vi "Drivetrain Control.vi"(0 "Back Left DevRef In":T1={"DeviceStatus"={"status"=FALSE, "code"=0, "source"=""}, "Type"=enum."PWM", "PWM"={"Digital Module"=enum."Digital Module 1", "PWM Channel"=enum."Invalid", "DeadBand"={"Name"="", "maxPositivePwm"=0, "minPositivePwm"=0, "centerPwm"=0, "maxNegativePwm"=0, "minNegativePwm"=0, "angularRange"=0}}, "CAN"={"Device Number"=0, "Control Mode"=enum."Percent VBus", "Semaphore"=refnum, "Max Vout"=12.0}, "Invert"=FALSE, "TransformRef"=refnum, "InvTransformRef"=refnum}, 1 "X Axis":dbl, 2 "Y Axis":dbl, 5 "Back Right DevRef In":T1={"DeviceStatus"={"status"=FALSE, "code"=0, "source"=""}, "Type"=enum."PWM", "PWM"={"Digital Module"=enum."Digital Module 1", "PWM Channel"=enum."Invalid", "DeadBand"={"Name"="", "maxPositivePwm"=0, "minPositivePwm"=0, "centerPwm"=0, "maxNegativePwm"=0, "minNegativePwm"=0, "angularRange"=0}}, "CAN"={"Device Number"=0, "Control Mode"=enum."Percent VBus", "Semaphore"=refnum, "Max Vout"=12.0}, "Invert"=FALSE, "TransformRef"=refnum, "InvTransformRef"=refnum}, 7 "Front Left DevRef In":T1={"DeviceStatus"={"status"=FALSE, "code"=0, "source"=""}, "Type"=enum."PWM", "PWM"={"Digital Module"=enum."Digital Module 1", "PWM Channel"=enum."Invalid", "DeadBand"={"Name"="", "maxPositivePwm"=0, "minPositivePwm"=0, "centerPwm"=0, "maxNegativePwm"=0, "minNegativePwm"=0, "angularRange"=0}}, "CAN"={"Device Number"=0, "Control Mode"=enum."Percent VBus", "Semaphore"=refnum, "Max Vout"=12.0}, "Invert"=FALSE, "TransformRef"=refnum, "InvTransformRef"=refnum}, 9 "Front Right DevRef In":T1={"DeviceStatus"={"status"=FALSE, "code"=0, "source"=""}, "Type"=enum."PWM", "PWM"={"Digital Module"=enum."Digital Module 1", "PWM Channel"=enum."Invalid", "DeadBand"={"Name"="", "maxPositivePwm"=0, "minPositivePwm"=0, "centerPwm"=0, "maxNegativePwm"=0, "minNegativePwm"=0, "angularRange"=0}}, "CAN"={"Device Number"=0, "Control Mode"=enum."Percent VBus", "Semaphore"=refnum, "Max Vout"=12.0}, "Invert"=FALSE, "TransformRef"=refnum, "InvTransformRef"=refnum}, 11 "Closed Loop On/Off":bool, 12 "Drivetrain Reverse Button":bool, 13 "Trigger":bool) -> (3 "Left Motor Value":dbl, 4 "Back Left DevRef Out":T1={"DeviceStatus"={"status"=FALSE, "code"=0, "source"=""}, "Type"=enum."PWM", "PWM"={"Digital Module"=enum."Digital Module 1", "PWM Channel"=enum."Invalid", "DeadBand"={"Name"="", "maxPositivePwm"=0, "minPositivePwm"=0, "centerPwm"=0, "maxNegativePwm"=0, "minNegativePwm"=0, "angularRange"=0}}, "CAN"={"Device Number"=0, "Control Mode"=enum."Percent VBus", "Semaphore"=refnum, "Max Vout"=12.0}, "Invert"=FALSE, "TransformRef"=refnum, "InvTransformRef"=refnum}, 6 "Back Right DevRef Out":T1={"DeviceStatus"={"status"=FALSE, "code"=0, "source"=""}, "Type"=enum."PWM", "PWM"={"Digital Module"=enum."Digital Module 1", "PWM Channel"=enum."Invalid", "DeadBand"={"Name"="", "maxPositivePwm"=0, "minPositivePwm"=0, "centerPwm"=0, "maxNegativePwm"=0, "minNegativePwm"=0, "angularRange"=0}}, "CAN"={"Device Number"=0, "Control Mode"=enum."Percent VBus", "Semaphore"=refnum, "Max Vout"=12.0}, "Invert"=FALSE, "TransformRef"=refnum, "InvTransformRef"=refnum}, 8 "Front Left DevRef Out":T1={"DeviceStatus"={"status"=FALSE, "code"=0, "source"=""}, "Type"=enum."PWM", "PWM"={"Digital Module"=enum."Digital Module 1", "PWM Channel"=enum."Invalid", "DeadBand"={"Name"="", "maxPositivePwm"=0, "minPositivePwm"=0, "centerPwm"=0, "maxNegativePwm"=0, "minNegativePwm"=0, "angularRange"=0}}, "CAN"={"Device Number"=0, "Control Mode"=enum."Percent VBus", "Semaphore"=refnum, "Max Vout"=12.0}, "Invert"=FALSE, "TransformRef"=refnum, "InvTransformRef"=refnum}, 10 "Front Right DevRef Out":T1={"DeviceStatus"={"status"=FALSE, "code"=0, "source"=""}, "Type"=enum."PWM", "PWM"={"Digital Module"=enum."Digital Module 1", "PWM Channel"=enum."Invalid", "DeadBand"={"Name"="", "maxPositivePwm"=0, "minPositivePwm"=0, "centerPwm"=0, "maxNegativePwm"=0, "minNegativePwm"=0, "angularRange"=0}}, "CAN"={"Device Number"=0, "Control Mode"=enum."Percent VBus", "Semaphore"=refnum, "Max Vout"=12.0}, "Invert"=FALSE, "TransformRef"=refnum, "InvTransformRef"=refnum}, 14 "Right Motor Value":dbl)   [LabVIEW 2012]
uses:
  <vilib>/Rock Robotics/WPI/MotorControl/WPI_MotorControlDeviceRef.ctl
  <vilib>/Rock Robotics/SystemInterfaces/Typedef/FPGA_TypedefDigitalModule.ctl
  <vilib>/Rock Robotics/SystemInterfaces/DIO/FPGA_DIOPWMChannel.ctl
  <vilib>/Rock Robotics/WPI/PWM/WPI_PWMDeadband.ctl
  <vilib>/Rock Robotics/WPI/CAN/Jaguar/SubVIs/WPI_CANJaguar_ControlMode.ctl
  <vilib>/Rock Robotics/WPI/PWM/WPI_PWMTransform_ConPane.ctl
  <vilib>/Rock Robotics/WPI/CAN/Jaguar/SubVIs/WPI_CANJaguar_SpeedReference.ctl
  Robot Global Data.vi
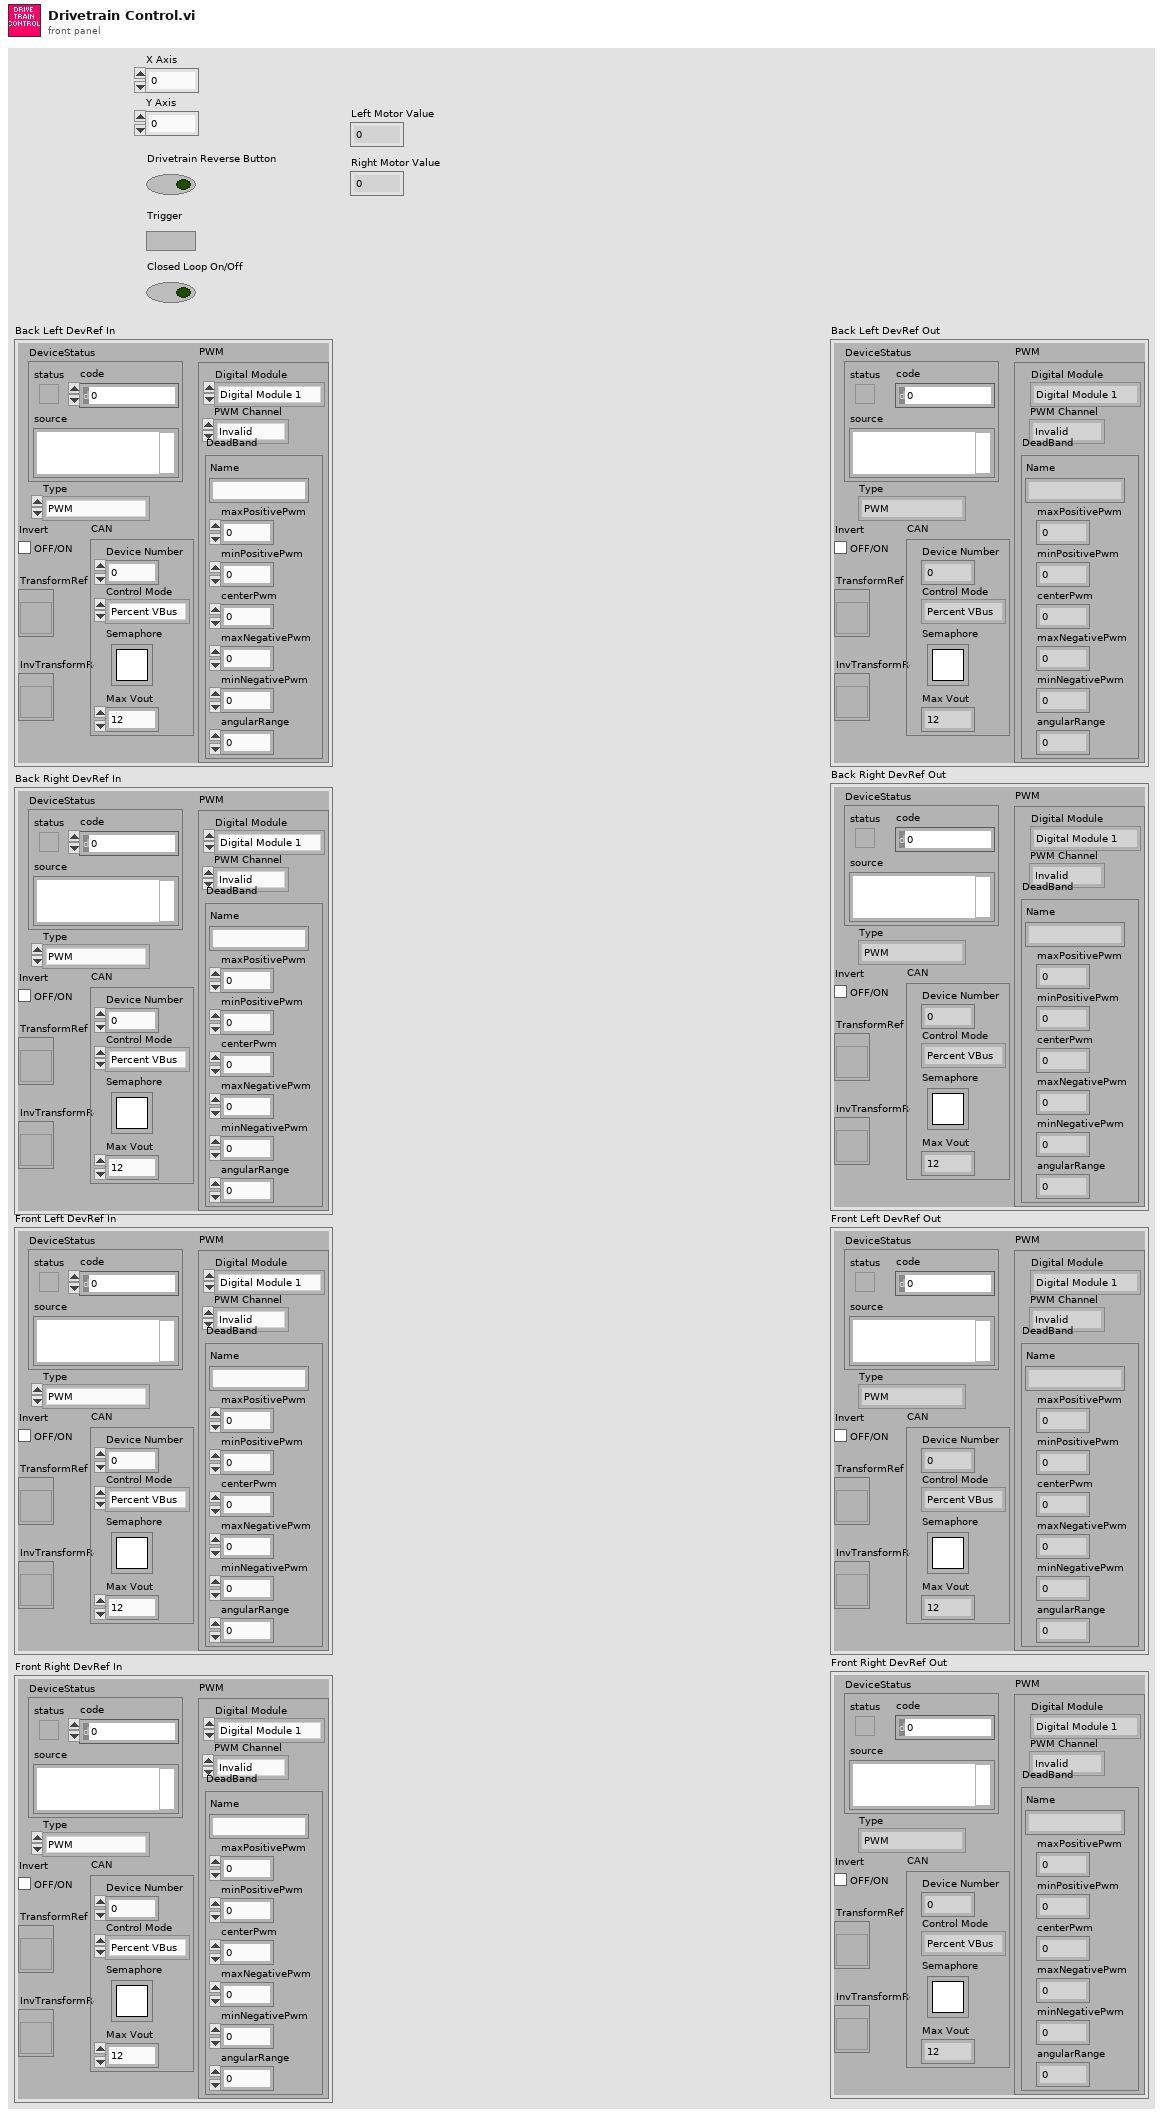
[diagram p1: front panel]
types:
  T1 = typedef "WPI_MotorControlDeviceRef.ctl" = cluster{"DeviceStatus":errorcluster, "Type":enum16{"PWM", "CAN"}, "PWM":cluster{"Digital Module":T2, "PWM Channel":T3, "DeadBand":T4}, "CAN":cluster{"Device Number":u8, "Control Mode":T5, "Semaphore":T6, "Max Vout":dbl}, "Invert":bool, "TransformRef":T7, "InvTransformRef":T7}
  T2 = typedef "FPGA_TypedefDigitalModule.ctl" = enum16{"Digital Module 1", "Digital Module 2"}
  T3 = typedef "FPGA_DIOPWMChannel.ctl" = enum8{"PWM 1", "PWM 2", "PWM 3", "PWM 4", "PWM 5", "PWM 6", "PWM 7", "PWM 8", "PWM 9", "PWM 10", "Invalid"}
  T4 = typedef "WPI_PWMDeadband.ctl" = cluster{"Name":string, "maxPositivePwm":i32, "minPositivePwm":i32, "centerPwm":i32, "maxNegativePwm":i32, "minNegativePwm":i32, "angularRange":u16}
  T5 = typedef "WPI_CANJaguar_ControlMode.ctl" = enum8{"Percent VBus", "Current", "Speed", "Position", "Voltage"}
  T6 = typedef "Semaphore RefNum" = refnum<k1>
  T7 = typedef "WPI_PWMTransform_ConPane.ctl" = refnum<vi>
  T8 = typedef "WPI_CANJaguar_SpeedReference.ctl" = u8
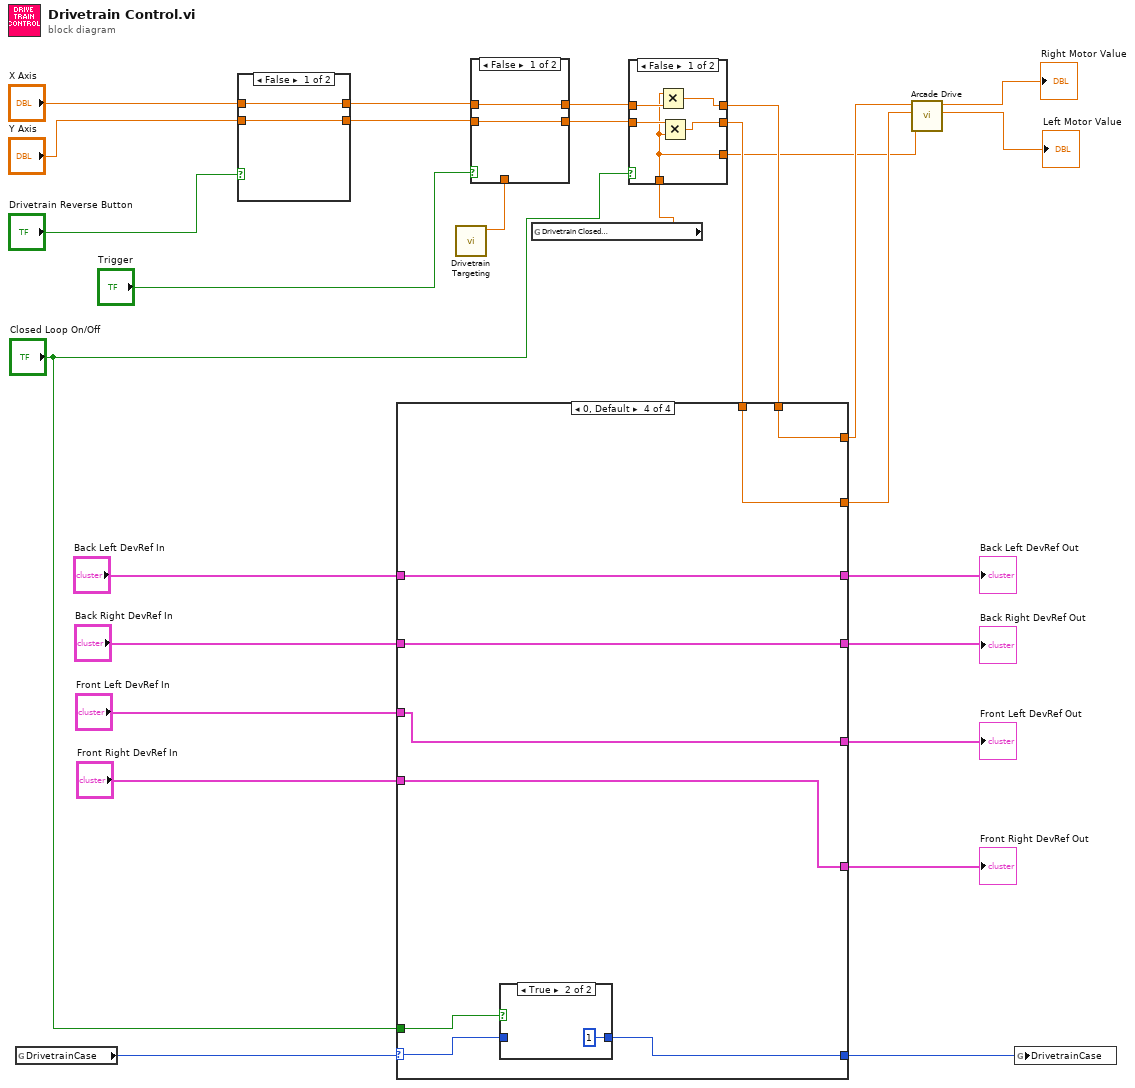
[diagram p0: block diagram]
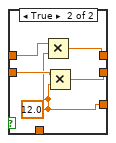
[diagram p2: hidden frame]
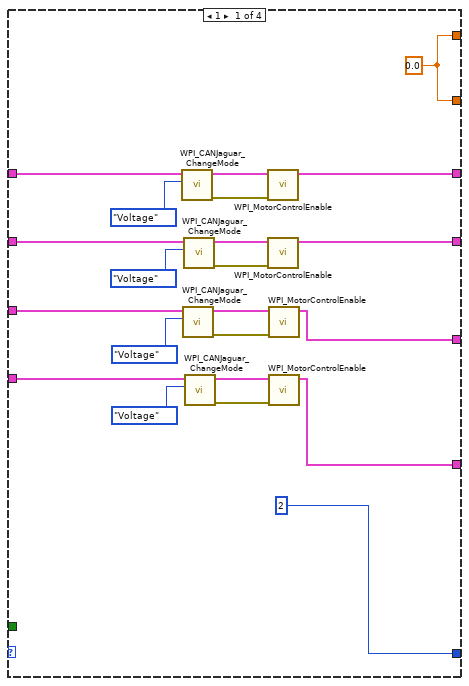
[diagram p3: hidden frame]
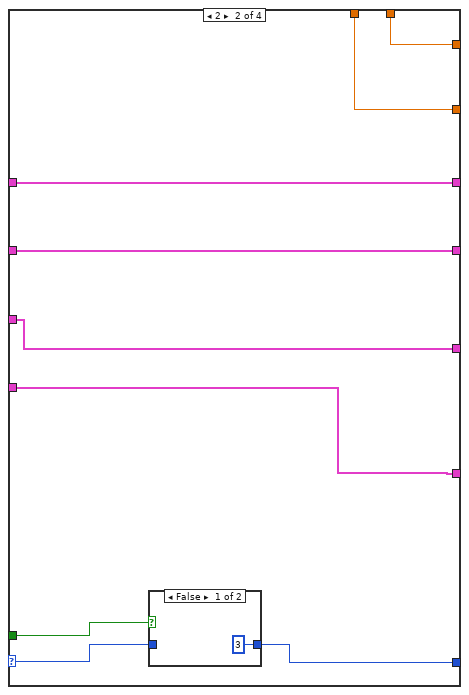
[diagram p4: hidden frame]
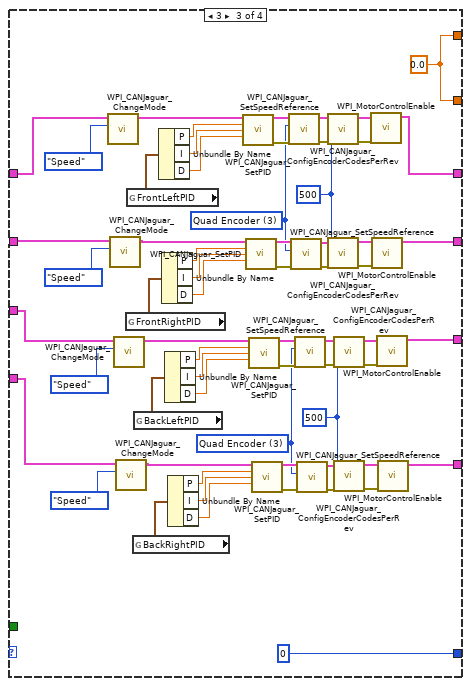
[diagram p6: hidden frame]
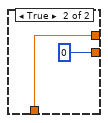
[diagram p8: hidden frame]
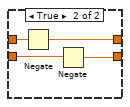
[diagram p9: hidden frame]
diagram:
  n1 = global read "Robot Global Data.vi" "DrivetrainCase"() -> (w20:i8)
  n2 = case shown="False" "Drivetrain Reverse Button" {
    tunnel: [w30 w31] -> w28
    tunnel: "X Axis" -> [w30 w34]
    tunnel: [w29 w32] -> w27
    tunnel: "Y Axis" -> [w29 w33]
    frame False {
    }
    frame True {
      n3 = Negate(x=w34) -> (-x=w31:dbl)
      n4 = Negate(x=w33) -> (-x=w32:dbl)
    }
  }
  n5 = call "Drivetrain Targeting.vi"() -> ("Drivetrain Center"=w23:dbl)  [unwired: 11 in]
  n6 = case shown="False" "Trigger" {
    tunnel: [w36 w37] -> w18
    tunnel: w28 -> [w36 _]
    tunnel: [w35 0] -> w17
    tunnel: w27 -> [w35 _]
    tunnel: w23 -> [_ w37]
    frame False {
    }
    frame True {
    }
  }
  n7 = global read "Robot Global Data.vi" "Drivetrain Closed\nLoop Max"() -> (w16:dbl)
  n8 = case shown="False" "Closed Loop On/Off" {
    tunnel: [w41 w46] -> w14
    tunnel: w18 -> [w43 w48]
    tunnel: [w40 w45] -> w15
    tunnel: w17 -> [w42 w47]
    tunnel: w16 -> [w39 _]
    tunnel: [w39 w44] -> w2
    frame False {
      n9 = Multiply(x=w39, y=w43) -> (x*y=w41:dbl)
      n10 = Multiply(x=w42, y=w39) -> (x*y=w40:dbl)
    }
    frame True {
      w44 = 12.0
      n11 = Multiply(x=w48, y=w44) -> (x*y=w46:dbl)
      n12 = Multiply(x=w47, y=w44) -> (x*y=w45:dbl)
    }
  }
  n13 = case shown="0, Default" w20 {
    selector: w20 -> [_ w76 _ w148]
    tunnel: [i8 2 ("ShooterCase") w75 i8 0 ("ShooterCase") w149] -> w19
    tunnel: "Back Left DevRef In" -> [w69 w79 w141 w152]
    tunnel: "Back Right DevRef In" -> [w68 w78 w140 w151]
    tunnel: [w61 w79 w113 w152] -> w6
    tunnel: [w60 w78 w114 w151] -> w5
    tunnel: "Closed Loop On/Off" -> [_ w77 _ w150]
    tunnel: w14 -> [_ w73 _ w147]
    tunnel: w15 -> [_ w74 _ w146]
    tunnel: [w59 w73 w112 w147] -> w13
    tunnel: [w59 w74 w112 w146] -> w12
    tunnel: "Front Left DevRef In" -> [w52 w72 w85 w145]
    tunnel: "Front Right DevRef In" -> [w51 w71 w84 w144]
    tunnel: [w50 w72 w83 w145] -> w4
    tunnel: [w49 w71 w82 w144] -> w3
    frame 1 {
      w59 = 0.0 ("FSpeed")
      n14 = call <vilib>:"WPI_CANJaguar_ChangeMode.vi"("Control Mode"=WPI_CANJaguar_ControlMode."Voltage", "CAN Jaguar Ref"=w69) -> ("error out"=w62:errorcluster, "CAN Jaguar Ref Out"=w63:T1)  [unwired: 8 in]
      n15 = call <vilib>:"WPI_CANJaguar_ChangeMode.vi"("Control Mode"=WPI_CANJaguar_ControlMode."Voltage", "CAN Jaguar Ref"=w52) -> ("error out"=w53:errorcluster, "CAN Jaguar Ref Out"=w54:T1)  [unwired: 8 in]
      n16 = call <vilib>:"WPI_CANJaguar_ChangeMode.vi"("Control Mode"=WPI_CANJaguar_ControlMode."Voltage", "CAN Jaguar Ref"=w68) -> ("error out"=w64:errorcluster, "CAN Jaguar Ref Out"=w65:T1)  [unwired: 8 in]
      n17 = call <vilib>:"WPI_CANJaguar_ChangeMode.vi"("Control Mode"=WPI_CANJaguar_ControlMode."Voltage", "CAN Jaguar Ref"=w51) -> ("error out"=w55:errorcluster, "CAN Jaguar Ref Out"=w56:T1)  [unwired: 8 in]
      n18 = call <vilib>:"WPI_MotorControlEnable.vi"("error in (no error)"=w62, "CAN Jaguar Ref"=w63) -> ("CAN Jaguar Ref Out"=w61:T1)  [unwired: 8 in, 1 out]
      n19 = call <vilib>:"WPI_MotorControlEnable.vi"("error in (no error)"=w64, "CAN Jaguar Ref"=w65) -> ("CAN Jaguar Ref Out"=w60:T1)  [unwired: 8 in, 1 out]
      n20 = call <vilib>:"WPI_MotorControlEnable.vi"("error in (no error)"=w53, "CAN Jaguar Ref"=w54) -> ("CAN Jaguar Ref Out"=w50:T1)  [unwired: 8 in, 1 out]
      n21 = call <vilib>:"WPI_MotorControlEnable.vi"("error in (no error)"=w55, "CAN Jaguar Ref"=w56) -> ("CAN Jaguar Ref Out"=w49:T1)  [unwired: 8 in, 1 out]
    }
    frame 2 {
      n22 = case shown="False" w77 {
        tunnel: [i8 3 ("ShooterCase") w81] -> w75
        tunnel: w76 -> [_ w81]
        frame False {
        }
        frame True {
        }
      }
    }
    frame 3 {
      w90 = u16 500 ("Encoder Codes Per Rev")
      w95 = T8 3 items=["Encoder"=0, "Inv Encoder"=2, "Quad Encoder"=3, "None"=255] ("Speed Reference")
      w112 = 0.0 ("FSpeed")
      w119 = u16 500 ("Encoder Codes Per Rev")
      w124 = T8 3 items=["Encoder"=0, "Inv Encoder"=2, "Quad Encoder"=3, "None"=255] ("Speed Reference")
      n23 = call <vilib>:"WPI_CANJaguar_ChangeMode.vi"("Control Mode"=WPI_CANJaguar_ControlMode."Speed", "CAN Jaguar Ref"=w141) -> ("CAN Jaguar Ref Out"=w139:T1)  [unwired: 8 in, 1 out]
      n24 = call <vilib>:"WPI_CANJaguar_ChangeMode.vi"("Control Mode"=WPI_CANJaguar_ControlMode."Speed", "CAN Jaguar Ref"=w140) -> ("CAN Jaguar Ref Out"=w130:T1)  [unwired: 8 in, 1 out]
      n25 = call <vilib>:"WPI_CANJaguar_ChangeMode.vi"("Control Mode"=WPI_CANJaguar_ControlMode."Speed", "CAN Jaguar Ref"=w85) -> ("CAN Jaguar Ref Out"=w109:T1)  [unwired: 8 in, 1 out]
      n26 = call <vilib>:"WPI_CANJaguar_ChangeMode.vi"("Control Mode"=WPI_CANJaguar_ControlMode."Speed", "CAN Jaguar Ref"=w84) -> ("CAN Jaguar Ref Out"=w100:T1)  [unwired: 8 in, 1 out]
      n27 = global read "Robot Global Data.vi" "FrontRightPID"() -> (w134:cluster{"P":dbl, "I":dbl, "D":dbl})
      n28 = global read "Robot Global Data.vi" "FrontLeftPID"() -> (w138:cluster{"P":dbl, "I":dbl, "D":dbl})
      n29 = global read "Robot Global Data.vi" "BackRightPID"() -> (w104:cluster{"P":dbl, "I":dbl, "D":dbl})
      n30 = global read "Robot Global Data.vi" "BackLeftPID"() -> (w108:cluster{"P":dbl, "I":dbl, "D":dbl})
      n31 = Unbundle By Name(w138) -> ("P"=w137:dbl, "I"=w136:dbl, "D"=w135:dbl)
      n32 = Unbundle By Name(w134) -> ("P"=w133:dbl, "I"=w132:dbl, "D"=w131:dbl)
      n33 = Unbundle By Name(w108) -> ("P"=w107:dbl, "I"=w106:dbl, "D"=w105:dbl)
      n34 = Unbundle By Name(w104) -> ("P"=w103:dbl, "I"=w102:dbl, "D"=w101:dbl)
      n35 = call <vilib>:"WPI_CANJaguar_SetPID.vi"("CAN Jaguar Ref"=w139, "P"=w137, "I"=w136, "D"=w135) -> ("CAN Jaguar Ref Out"=w127:T1, "error out"=w128:errorcluster)  [unwired: 10 in]
      n36 = call <vilib>:"WPI_CANJaguar_SetPID.vi"("CAN Jaguar Ref"=w130, "P"=w133, "I"=w132, "D"=w131) -> ("CAN Jaguar Ref Out"=w126:T1, "error out"=w125:errorcluster)  [unwired: 10 in]
      n37 = call <vilib>:"WPI_CANJaguar_SetPID.vi"("CAN Jaguar Ref"=w109, "P"=w107, "I"=w106, "D"=w105) -> ("CAN Jaguar Ref Out"=w98:T1, "error out"=w99:errorcluster)  [unwired: 10 in]
      n38 = call <vilib>:"WPI_CANJaguar_SetPID.vi"("CAN Jaguar Ref"=w100, "P"=w103, "I"=w102, "D"=w101) -> ("CAN Jaguar Ref Out"=w97:T1, "error out"=w96:errorcluster)  [unwired: 10 in]
      n39 = call <vilib>:"WPI_CANJaguar_SetSpeedReference.vi"("error in (no error)"=w128, "Speed Reference"=w124, "CAN Jaguar Ref"=w127) -> ("error out"=w123:errorcluster, "CAN Jaguar Ref Out"=w122:T1)  [unwired: 7 in]
      n40 = call <vilib>:"WPI_CANJaguar_SetSpeedReference.vi"("error in (no error)"=w125, "Speed Reference"=w124, "CAN Jaguar Ref"=w126) -> ("error out"=w120:errorcluster, "CAN Jaguar Ref Out"=w121:T1)  [unwired: 7 in]
      n41 = call <vilib>:"WPI_CANJaguar_SetSpeedReference.vi"("error in (no error)"=w99, "Speed Reference"=w95, "CAN Jaguar Ref"=w98) -> ("error out"=w94:errorcluster, "CAN Jaguar Ref Out"=w93:T1)  [unwired: 7 in]
      n42 = call <vilib>:"WPI_CANJaguar_SetSpeedReference.vi"("error in (no error)"=w96, "Speed Reference"=w95, "CAN Jaguar Ref"=w97) -> ("error out"=w91:errorcluster, "CAN Jaguar Ref Out"=w92:T1)  [unwired: 7 in]
      n43 = call <vilib>:"WPI_CANJaguar_ConfigEncoderCodesPerRev.vi"("error in (no error)"=w123, "Encoder Codes Per Rev"=w119, "CAN Jaguar Ref"=w122) -> ("error out"=w118:errorcluster, "CAN Jaguar Ref Out"=w117:T1)  [unwired: 7 in]
      n44 = call <vilib>:"WPI_CANJaguar_ConfigEncoderCodesPerRev.vi"("error in (no error)"=w120, "Encoder Codes Per Rev"=w119, "CAN Jaguar Ref"=w121) -> ("error out"=w116:errorcluster, "CAN Jaguar Ref Out"=w115:T1)  [unwired: 7 in]
      n45 = call <vilib>:"WPI_CANJaguar_ConfigEncoderCodesPerRev.vi"("error in (no error)"=w94, "Encoder Codes Per Rev"=w90, "CAN Jaguar Ref"=w93) -> ("error out"=w89:errorcluster, "CAN Jaguar Ref Out"=w88:T1)  [unwired: 7 in]
      n46 = call <vilib>:"WPI_CANJaguar_ConfigEncoderCodesPerRev.vi"("error in (no error)"=w91, "Encoder Codes Per Rev"=w90, "CAN Jaguar Ref"=w92) -> ("error out"=w87:errorcluster, "CAN Jaguar Ref Out"=w86:T1)  [unwired: 7 in]
      n47 = call <vilib>:"WPI_MotorControlEnable.vi"("error in (no error)"=w118, "CAN Jaguar Ref"=w117) -> ("CAN Jaguar Ref Out"=w113:T1)  [unwired: 8 in, 1 out]
      n48 = call <vilib>:"WPI_MotorControlEnable.vi"("error in (no error)"=w116, "CAN Jaguar Ref"=w115) -> ("CAN Jaguar Ref Out"=w114:T1)  [unwired: 8 in, 1 out]
      n49 = call <vilib>:"WPI_MotorControlEnable.vi"("error in (no error)"=w89, "CAN Jaguar Ref"=w88) -> ("CAN Jaguar Ref Out"=w83:T1)  [unwired: 8 in, 1 out]
      n50 = call <vilib>:"WPI_MotorControlEnable.vi"("error in (no error)"=w87, "CAN Jaguar Ref"=w86) -> ("CAN Jaguar Ref Out"=w82:T1)  [unwired: 8 in, 1 out]
    }
    frame 0, Default {
      n51 = case shown="True" w150 {
        tunnel: [w153 i8 1 ("ShooterCase")] -> w149
        tunnel: w148 -> [w153 _]
        frame False {
        }
        frame True {
        }
      }
    }
  }
  "Back Left DevRef Out" <- w6
  "Back Right DevRef Out" <- w5
  "Front Left DevRef Out" <- w4
  "Front Right DevRef Out" <- w3
  n52 = call "Arcade Drive.vi"("Max Output"=w2, "Y Axis"=w12, "X Axis"=w13) -> ("Left Motor Value"=→"Left Motor Value":dbl, "Right Motor Value"=→"Right Motor Value":dbl)  [unwired: 7 in]
  n53 = global write "Robot Global Data.vi" "DrivetrainCase"(w19) -> ()
